vi "SCMP - System init.vi"(8 "error in (no error)":errorcluster, 9 "Pane Color":u32, 10 "instrument":string) -> (0 "error main":errorcluster, 1 "Andor array":T1[](array[typedef]) {"Exposure (s)" format="%^.3g"; "Time at Synch" format="%<%H:%M:%S>T"; "Interframe Time" format="%#_3g"; "Frame Readout Time" format="%_3g"; "Row Readout Time" format="%_3g"}, 2 "Peripherals":T4, 3 "cont?":bool=TRUE, 5 "Today's SCMP Engineering File":path, 7 "version":string)   [LabVIEW 2014]
uses:
  Controls/Global demo.vi
  AISAS/Controls/focus.ctl
  Controls/CoMP-S Controls/Emission Line Filter Wheel.ctl
  Controls/CoMP-S Controls/Polarization Optics Filter Wheel.ctl
  Controls/SCD - EDT - Emission Line Filter Wheel.ctl
  Controls/SCD - Calibration Optics Filter Wheel.ctl
  AISAS/Controls/Diffuser.ctl
  Controls/SCD - FITS Cluster.ctl
  Controls/Globals.vi
  AISAS/Mech/AISAS Mech.lvclass
  Controls/peripherals.ctl
  Controls/Cameras select.ctl
  Camera/Andor Neo Info.ctl
  Controls/beaning.ctl
panel:
  in  "Force PI Init":bool
  in  "Shutter":string(combo)="Global"
  in  "Temperature":string(combo)="-25.00"
  out "Andor 2":T1={"Handle"=0, "Pixel Encoding"="", "AOI Width"=0, "AOI Height"=0, "AOI Stride"=0, "Row Readout Time"=0.0, "Frame Readout Time"=0.0, "Interframe Time"=0.0, "Semaphore"=refnum, "SerialNumber"="", "Camera Model"="", "Controller ID"="", "Firmware Version"="", "Shutter"="Global", "BDiv"=1, "Time at Synch"=timestamp(3029526000.379448 s since 1904-01-01), "Idx"=0, "PreAmp"="", "Binning"=enum."1x1", "PixelReadoutRate"="", "Exposure (s)"=0.05, "Image Bytes"=0, "Image Pixels"=0, "SpuriousNoiseFilter"=FALSE, "Overlap"=FALSE, "CycleMode"=""} {"Exposure (s)" format="%^.3g"; "Time at Synch" format="%<%H:%M:%S>T"; "Interframe Time" format="%#_3g"; "Frame Readout Time" format="%_3g"; "Row Readout Time" format="%_3g"}
  out "Timestamp at Synch 2":timestamp
  out "error eng":errorcluster
  out "Andor 1":T1={"Handle"=0, "Pixel Encoding"="", "AOI Width"=0, "AOI Height"=0, "AOI Stride"=0, "Row Readout Time"=0.0, "Frame Readout Time"=0.0, "Interframe Time"=0.0, "Semaphore"=refnum, "SerialNumber"="", "Camera Model"="", "Controller ID"="", "Firmware Version"="", "Shutter"="Global", "BDiv"=1, "Time at Synch"=timestamp(3029526000.379448 s since 1904-01-01), "Idx"=0, "PreAmp"="", "Binning"=enum."1x1", "PixelReadoutRate"="", "Exposure (s)"=0.05, "Image Bytes"=0, "Image Pixels"=0, "SpuriousNoiseFilter"=FALSE, "Overlap"=FALSE, "CycleMode"=""} caption="Andor1" {"Exposure (s)" format="%^.3g"; "Time at Synch" format="%<%H:%M:%S>T"; "Interframe Time" format="%#_3g"; "Frame Readout Time" format="%_3g"; "Row Readout Time" format="%_3g"}
  out "Timestamp at Synch":timestamp
  # "System initialization\n        wait please"
  # "Peripherals"
  # "Andor control"
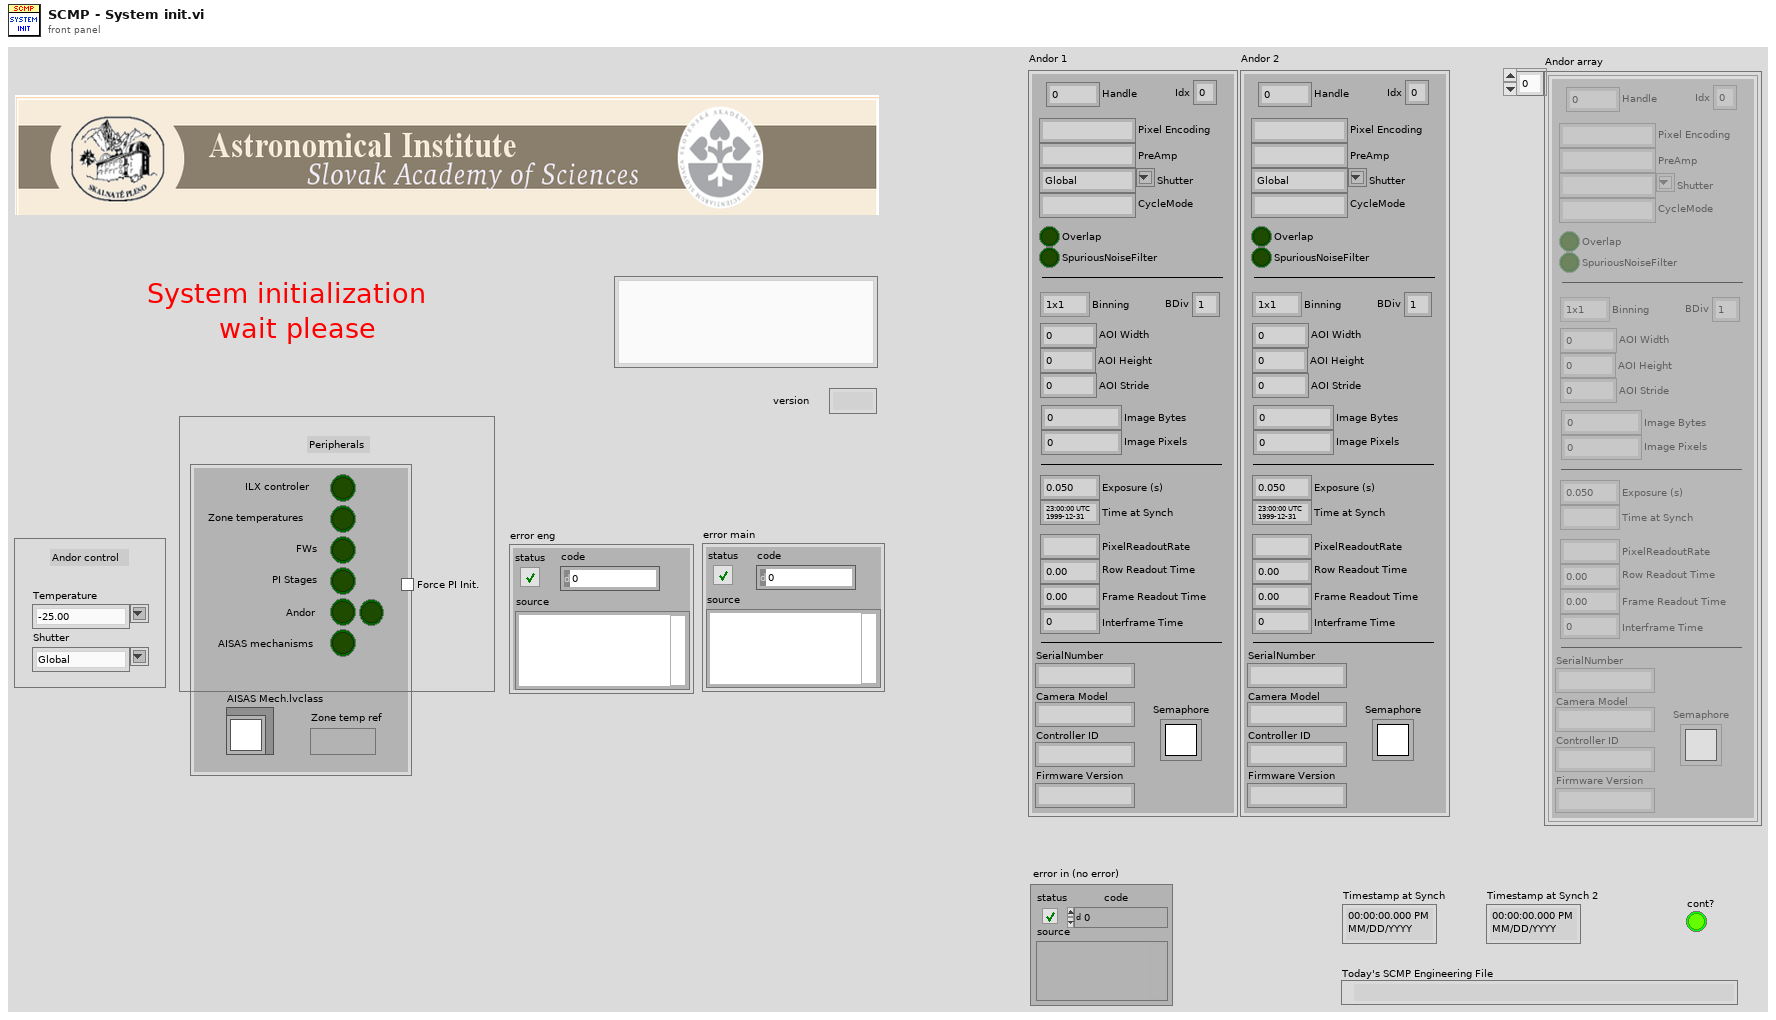
[diagram p1: front panel]
types:
  T1 = typedef "Andor Neo Info.ctl" = cluster{"Handle":i32, "Pixel Encoding":string, "AOI Width":i32, "AOI Height":i32, "AOI Stride":i32, "Row Readout Time":dbl, "Frame Readout Time":dbl, "Interframe Time":dbl, "Semaphore":T2, "SerialNumber":string, "Camera Model":string, "Controller ID":string, "Firmware Version":string, "Shutter":string, "BDiv":u8, "Time at Synch":timestamp, "Idx":i32, "PreAmp":string, "Binning":T3, "PixelReadoutRate":string, "Exposure (s)":dbl, "Image Bytes":i64, "Image Pixels":i64, "SpuriousNoiseFilter":bool, "Overlap":bool, "CycleMode":string}
  T2 = typedef "Semaphore RefNum" = refnum<k1>
  T3 = typedef "beaning.ctl" = enum16{"1x1", "2x2", "3x3", "4x4", "8x8"}
  T4 = typedef "peripherals.ctl" = cluster{"ILX controler":bool, "Zone temperatures":bool, "Andor":bool, "Andor 2":bool, "PI Stages":bool, "AISAS mechanisms":bool, "AISAS Mech.lvclass":refnum<class "AISAS Mech.lvclass">, "Zone temp ref":variant, "FWs":bool}
  T5 = cluster{"server address":string, "remote port (502)":u16}
  T6 = enum32{"Invalid", "Standard", "Closed", "Hidden", "Minimized", "Maximized"}
  T7 = typedef "SCD - FITS Cluster.ctl" = cluster{"Wavelength (nm)":dbl, "Exposure (s)":dbl, "Tuning Delay (ms)":dbl, "Beam Type (-1/1)":dbl, "Tuning Voltages":dbl[], "Observer":string, "Light Shapping Diffuser":T8, "Comment":string, "Data Type":u16, "Mod Cycles":u16, "SCD Calibration Optics":T9, "SCD Emission Line Filter":T10, "Cookbook":string, "COMP-S Calibration Wheel":T11, "COMP-S Andover Filter Wheel":T12, "FOV Rotation (deg)":dbl, "Objective Lens Position (mm)":T13, "Occulter size":dbl, "Time End":timestamp, "Acc Exposure (s)":dbl, "Time Stamp Array":timestamp[], "Camera Serial Number":string[], "Camera Temp":dbl[], "Camera PI (mm)":dbl[], "Time Start":timestamp, "Peripherals":T4, "FITS paths":path[], "Cameras":T14, "load preset cbk":bool, "periodic check count":i32, "COMP-S Calibration Wheel 2":T11, "Calib":enum16{"Dark", "Flat"}, "Abso Aperture":dbl, "Nominal Aperture":dbl}
  T8 = typedef "Diffuser.ctl" = enum16{"Out of Beam", "In Beam"}
  T9 = typedef "SCD - Calibration Optics Filter Wheel.ctl" = enum16{"1 - Polarizer @0, I+Q", "2 - Polarizer @90, I-Q", "3 - Polarizer @45, I+U", "4 - Polarizer @135, I-U", "5 - Polarizer @0, Retarder @45, I+V", "6 - Polarizer @0, Retarder @135, I-V", "7 - Dark", "8 - Clear", "9 - N/A"}
  T10 = typedef "SCD - EDT - Emission Line Filter Wheel.ctl" = enum16{"1-557.6nm", "2-587.6nm", "3-589.6nm", "4-630.2nm", "5-656.4nm", "6-849.8nm", "7-854.2nm", "8-866.2nm", "9-1083.0nm"}
  T11 = typedef "Polarization Optics Filter Wheel.ctl" = enum16{"Dark", "Clear", "Exchange Lens", "Polarizer @0, I+Q", "Polarizer @90, I-Q", "Polarizer @45, I+U", "Polarizer @135, I-U", "Polarizer @0, Retarder @45, I+V", "Polarizer @0, Retarder @135, I-V"}
  T12 = typedef "Emission Line Filter Wheel.ctl" = enum16{"530.3nm/HWB 0.34nm (Fe XIV)", "587.6nm/HBW 0.44nm (He I D3)", "637.5nm/HBW 0.53nm (Fe X)", "656.3nm/HBW 0.57nm (H-Alpha)", "789.2nm/HBW 0.85nm (Fe XI)", "854.2nm/HBW 1.01nm (Ca I)", "1074.7nm/HBW 2.34nm (Fe XIII)", "1079.8nm/HBW 1.64nm (Fe XIII)", "1083.0nm/HBW 1.66nm (He I)"}
  T13 = typedef "focus.ctl" = dbl
  T14 = typedef "Cameras select.ctl" = enum16{"Andor", "GDR"}
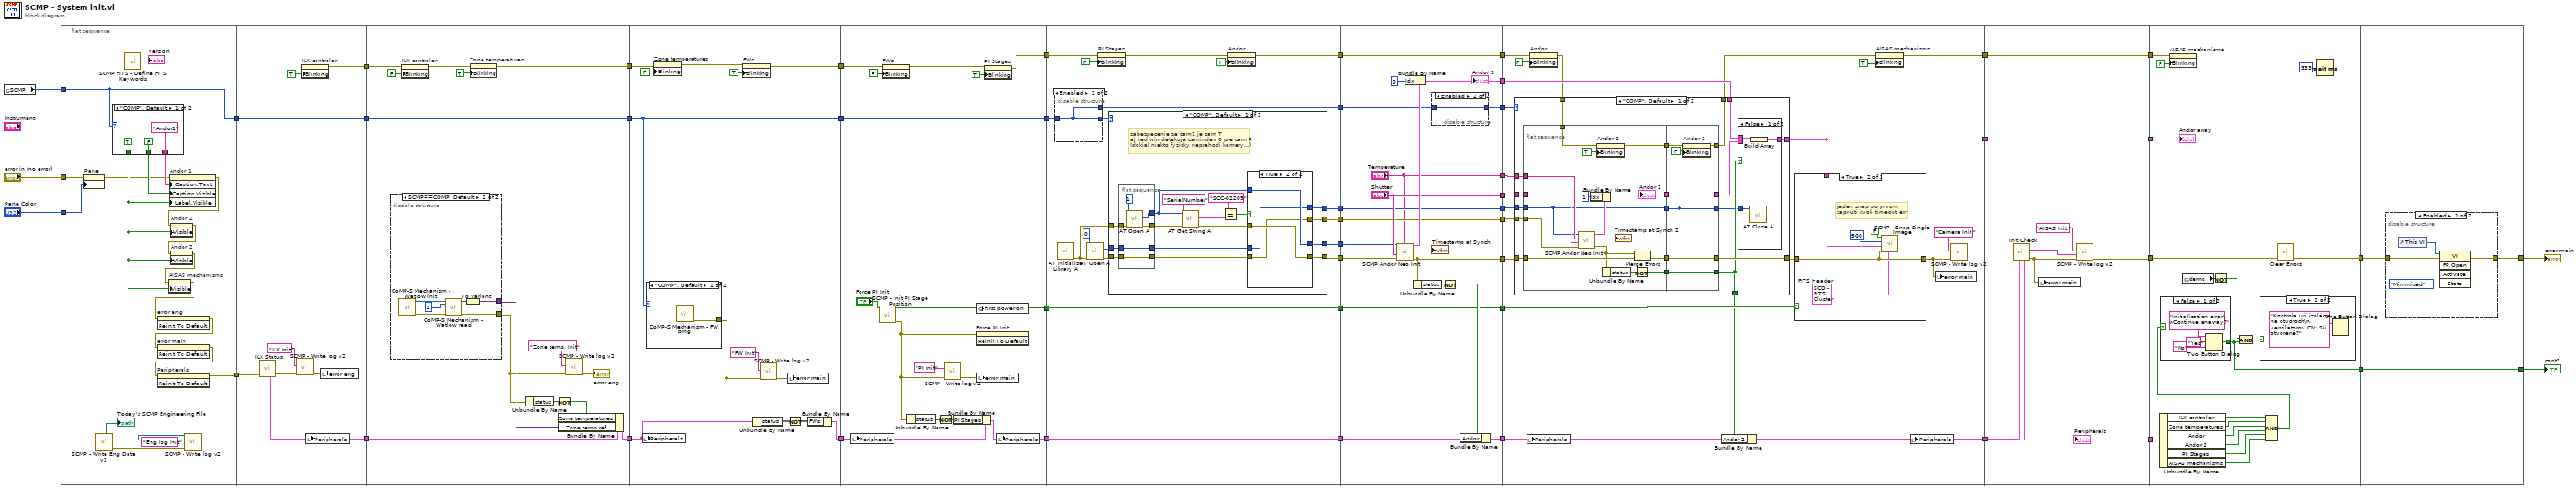
[diagram p0: block diagram]
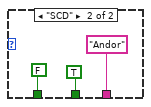
[diagram p2: hidden frame]
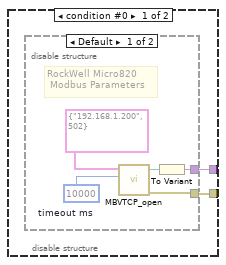
[diagram p3: hidden frame]
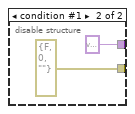
[diagram p4: hidden frame]
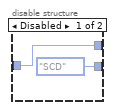
[diagram p6: hidden frame]
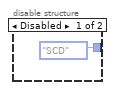
[diagram p9: hidden frame]
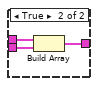
[diagram p10: hidden frame]
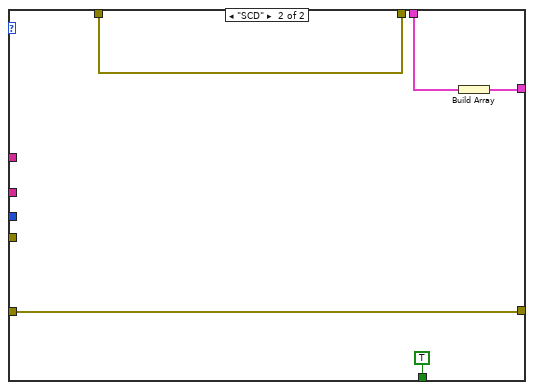
[diagram p11: hidden frame]
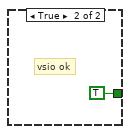
[diagram p14: hidden frame]
diagram:
  n1 = global read "Globals.vi" "SCMP"() -> (w11:enum16{"COMP", "SCD"})
  n2 = flat-sequence {
    tunnel: [w61] -> w38
    tunnel: [w53] -> w19
    tunnel: "error in (no error)" -> [w56]
    tunnel: "Pane Color" -> [w54]
    tunnel: w11 -> [w53]
    tunnel: [w73] -> w8
    tunnel: [w79] -> w7
    tunnel: w38 -> [w78]
    tunnel: w19 -> [w77]
    tunnel: [w77] -> w6
    tunnel: w8 -> [w92]
    tunnel: [w91] -> w41
    tunnel: [w89] -> w39
    tunnel: [w87] -> w16
    tunnel: w6 -> [w87]
    tunnel: w7 -> [w85]
    tunnel: w41 -> [w115]
    tunnel: [w116] -> w40
    tunnel: w39 -> [w120]
    tunnel: [w114] -> w17
    tunnel: w16 -> [w114]
    tunnel: [w117] -> w5
    tunnel: w40 -> [w130]
    tunnel: [w136] -> w29
    tunnel: [w131] -> w18
    tunnel: w17 -> [w131]
    tunnel: w5 -> [w127]
    tunnel: [w125] -> w4
    tunnel: [w123] -> w3
    tunnel: [w143] -> w37
    tunnel: [w152] -> w36
    tunnel: [w149] -> w33
    tunnel: [w148] -> w32
    tunnel: [w147] -> w31
    tunnel: [w146] -> w30
    tunnel: w29 -> [w144]
    tunnel: [w144] -> w28
    tunnel: w18 -> [w139]
    tunnel: w4 -> [w141]
    tunnel: w3 -> [w143]
    tunnel: [w138] -> w2
    tunnel: [w209] -> w47
    tunnel: [w201] -> w46
    tunnel: [w206] -> w45
    tunnel: ["Shutter"] -> w44
    tunnel: ["Temperature"] -> w43
    tunnel: w37 -> [w204]
    tunnel: [w200] -> w42
    tunnel: w36 -> [w200]
    tunnel: [w196] -> w35
    tunnel: [w197] -> w34
    tunnel: w33 -> [w199]
    tunnel: w32 -> [w198]
    tunnel: w31 -> [w197]
    tunnel: w30 -> [w196]
    tunnel: w28 -> [w195]
    tunnel: [w195] -> w27
    tunnel: [w192] -> w15
    tunnel: w2 -> [w191]
    tunnel: w47 -> [w232]
    tunnel: w46 -> [w222]
    tunnel: [w219] -> w24
    tunnel: w45 -> [w228]
    tunnel: w44 -> [w230]
    tunnel: w43 -> [w229]
    tunnel: w42 -> [w227]
    tunnel: [w221] -> w23
    tunnel: w35 -> [w225]
    tunnel: w34 -> [w224]
    tunnel: w27 -> [w223]
    tunnel: [w214] -> w20
    tunnel: w15 -> [w212]
    tunnel: [w297] -> w25
    tunnel: w24 -> [w292]
    tunnel: w23 -> [w298]
    tunnel: [w298] -> w22
    tunnel: [w296] -> w21
    tunnel: w20 -> [w296]
    tunnel: [w291] -> w14
    tunnel: w25 -> [w300]
    tunnel: w22 -> [w315]
    tunnel: w21 -> [w313]
    tunnel: w14 -> [w301]
    tunnel: [w299] -> w10
    tunnel: [w304] -> w9
    tunnel: [w325] -> w26
    tunnel: w10 -> [w324]
    tunnel: w9 -> [w325]
    tunnel: [w323] -> w1
    frame #0 {
      n3 = property on="Pane" class="Pane"(error in=w56, "PaneColor"=w54) -> (error out=w55:errorcluster)  [unwired: 1 in, 1 out]
      n4 = call "SCMP - Write Eng Data v2.vi"() -> ("error out"=w48:errorcluster, "Today's SCMP folder"=w51:path, "Today's SCMP Engineering File"=→"Today's SCMP Engineering File":path)  [unwired: 8 in, 1 out]
      n5 = case shown="\"COMP\", Default" w53 {
        tunnel: ["Andor1" ("Caption.Text") "Andor" ("Caption.Text")] -> w66
        tunnel: [FALSE ("Caption.Visible") TRUE ("Caption.Visible")] -> w65
        tunnel: [TRUE ("Caption.Visible") FALSE ("Caption.Visible")] -> w58
        frame "COMP", Default {
        }
        frame "SCD" {
        }
      }
      n6 = call "SCMP FITS - Define FITS Keywords.vi"() -> ("Version"=→"version":string)  [unwired: 5 in, 6 out]
      n7 = property on="Andor 1" class="Clust (strict)"(error in=w55, "Caption.Text"=w66, "Caption.Visible"=w65, "Label.Visible"=w58) -> (error out=w64:errorcluster)  [unwired: 1 in, 1 out]
      n8 = property on="Andor 2" class="Clust (strict)"(error in=w64, "Visible"=w58) -> (error out=w60:errorcluster)  [unwired: 1 in, 1 out]
      n9 = property on="Andor 2" class="Bool (strict)"(error in=w60, "Visible"=w58) -> (error out=w59:errorcluster)  [unwired: 1 in, 1 out]
      n10 = property on="AISAS mechanisms" class="Bool (strict)"(error in=w59, "Visible"=w58) -> (error out=w57:errorcluster)  [unwired: 1 in, 1 out]
      n11 = invoke on="error eng" class="Clust (strict)" method="Reinit To Default"(error in=w57) -> (error out=w63:errorcluster)  [unwired: 2 in, 2 out]
      n12 = invoke on="error main" class="Clust (strict)" method="Reinit To Default"(error in=w63) -> (error out=w62:errorcluster)  [unwired: 2 in, 2 out]
      n13 = invoke on="Peripherals" class="Clust (strict)" method="Reinit To Default"(error in=w62) -> (error out=w61:errorcluster)  [unwired: 2 in, 2 out]
      n14 = call "SCMP - Write log v2.vi"("Error to log"=w48, "data"="Eng log Init" ("mesage"), "Today's SCMP folder"=w51) -> ()  [unwired: 6 in, 3 out]
    }
    frame #1 {
      n15 = call "ILX Status.vi"("error in"=w78) -> ("error out"=w76:errorcluster, "Peripherals out"=w73:T4)  [unwired: 5 in, 4 out]
      n16 = call "SCMP - Write log v2.vi"("Error to log"=w76, "data"="ILX Init" ("mesage")) -> ("error out"=w74:errorcluster)  [unwired: 7 in, 2 out]
      n17 = property on="ILX controler" class="Bool (strict)"("Blinking"=TRUE) -> (error out=w79:errorcluster)  [unwired: 2 in, 1 out]
      n18 = local write "Peripherals"(w73) -> ()
      n19 = local write "error eng"(w74) -> ()
    }
    frame #2 {
      n20 = disable-structure shown="SCMP==COMP, Default" {
        disable-tunnel: [w96 w104] -> w82
        disable-tunnel: [w95 w105] -> w88
        frame condition #0 {
          n21 = disable-structure shown="Default" {
            disable-tunnel: [w97 errorcluster {"status"=FALSE, "code"=0, "source"=""} ("error in")] -> w96
            disable-tunnel: [w98 variant ("Variant")] -> w95
            frame condition #0 (active) {
              w100 = 10000  # timeout ms
              # "RockWell Micro820\n Modbus Parameters"
              n22 = call <vilib>:"MBVTCP_open.vi"("timeout ms (60000)"=w100, "Network"=T5 {"server address"="192.168.1.200", "remote port (502)"=502} ("Rockwell Address and Port")) -> ("error out"=w97:errorcluster, "NetRefTCP out"=w99:refnum<k5>)  [unwired: 1 in, 7 out]
              n23 = To Variant(anything=w99) -> (Variant=w98:variant)
            }
            frame condition #1 {
            }
          }
        }
        frame condition #1 (active) {
          n24 = call "CoMP-S Mechanism - Watlow init.vi"() -> ("error out"=w106:errorcluster, "ILabVIEW"=w107:refnum<k24>)  [unwired: 8 in, 1 out]
          n25 = call "CoMP-S Mechanism - Watlow read.vi"("6. Instance ID"=1, "error in (no error)"=w106, "ILabVIEW In"=w107) -> ("error out"=w104:errorcluster)  [unwired: 4 in, 2 out]
          n26 = To Variant(anything=w107) -> (Variant=w105:variant)
        }
      }
      n27 = property on="ILX controler" class="Bool (strict)"(error in=w85, "Blinking"=FALSE) -> (error out=w84:errorcluster)  [unwired: 1 in, 1 out]
      n28 = property on="Zone temperatures" class="Bool (strict)"(error in=w84, "Blinking"=TRUE) -> (error out=w89:errorcluster)  [unwired: 1 in, 1 out]
      n29 = Unbundle By Name(w82) -> ("status"=w94:bool)
      n30 = Not(x=w94) -> (.not. x?=w90:bool)
      n31 = Bundle By Name(cluster=w92, "Zone temperatures"=w90, "Zone temp ref"=w88) -> (w91:T4)
      n32 = call "SCMP - Write log v2.vi"("Error to log"=w82, "data"="Zone temp. Init" ("mesage")) -> ("error out"=→"error eng":errorcluster)  [unwired: 7 in, 2 out]
    }
    frame #3 {
      n33 = local write "Peripherals"(w115) -> ()
      n34 = case shown="\"COMP\", Default" w114 {
        tunnel: [w122 _] -> w111
        frame "COMP", Default {
          n35 = call "CoMP-S Mechanism - FW ping.vi"() -> ("error out"=w122:errorcluster)  [unwired: 10 in, 1 out]
        }
        frame "SCD" {
        }
      }
      n36 = property on="Zone temperatures" class="Bool (strict)"(error in=w120, "Blinking"=FALSE) -> (error out=w118:errorcluster)  [unwired: 1 in, 1 out]
      n37 = property on="FWs" class="Bool (strict)"(error in=w118, "Blinking"=TRUE) -> (error out=w117:errorcluster)  [unwired: 1 in, 1 out]
      n38 = Unbundle By Name(w111) -> ("status"=w113:bool)
      n39 = call "SCMP - Write log v2.vi"("Error to log"=w111, "data"="FW Init" ("mesage")) -> ("error out"=w109:errorcluster)  [unwired: 7 in, 2 out]
      n40 = Not(x=w113) -> (.not. x?=w112:bool)
      n41 = local write "error main"(w109) -> ()
      n42 = Bundle By Name(cluster=w115, "FWs"=w112) -> (w116:T4)
    }
    frame #4 {
      n43 = local write "Peripherals"(w130) -> ()
      n44 = call "SCMP - Init PI Stage Position.vi"("Force PI Init"="Force PI Init") -> ("error out"=w124:errorcluster, "first power on"=w136:bool)  [unwired: 9 in]
      n45 = property on="FWs" class="Bool (strict)"(error in=w127, "Blinking"=FALSE) -> (error out=w126:errorcluster)  [unwired: 1 in, 1 out]
      n46 = Unbundle By Name(w124) -> ("status"=w135:bool)
      n47 = Not(x=w135) -> (.not. x?=w134:bool)
      n48 = call "SCMP - Write log v2.vi"("Error to log"=w124, "data"="PI Init" ("mesage")) -> ("error out"=w132:errorcluster)  [unwired: 7 in, 2 out]
      n49 = Bundle By Name(cluster=w130, "PI Stages"=w134) -> (w123:T4)
      n50 = global write "Globals.vi" "first power on"(w136) -> ()
      n51 = invoke on="Force PI Init" class="Bool (strict)" method="Reinit To Default"(error in=w124) -> ()  [unwired: 2 in, 3 out]
      n52 = local write "error main"(w132) -> ()
      n53 = property on="PI Stages" class="Bool (strict)"(error in=w126, "Blinking"=TRUE) -> (error out=w125:errorcluster)  [unwired: 1 in, 1 out]
      n54 = local write "Peripherals"(w123) -> ()
    }
    frame #5 {
      n55 = disable-structure shown="Enabled" {
        disable-tunnel: [enum16{"COMP", "SCD"}."SCD" ("SCMP") w158] -> w140
        disable-tunnel: w139 -> [w156 w158]
        disable-tunnel: [w156 w158] -> w138
        frame Disabled {
        }
        frame Enabled {
        }
      }
      n56 = call <userlib>:"AT Initialise Library A.vi"() -> ("error out"=w142:errorcluster)  [unwired: 10 in, 1 out]
      n57 = call <userlib>:"AT Open A.vi"("error in (no error)"=w142, "CameraIndex"=0) -> ("error out"=w150:errorcluster, "Handle"=w145:i32)  [unwired: 7 in, 1 out]
      n58 = property on="PI Stages" class="Bool (strict)"(error in=w141, "Blinking"=FALSE) -> (error out=w155:errorcluster)  [unwired: 1 in, 1 out]
      n59 = case shown="\"COMP\", Default" w140 {
        tunnel: w150 -> [w174 w189]
        tunnel: [w173 w190] -> w149
        tunnel: [w172 w189] -> w148
        tunnel: [w171 _] -> w147
        tunnel: [w170 _] -> w146
        tunnel: w145 -> [w169 w190]
        tunnel: w142 -> [w168 _]
        frame "COMP", Default {
          # "zabezpecenie ze cam1 je cam T\naj ked win detekuje camindex 0 pre cam R\n(dokial niekto fyzicky neprehodi kamery...)"
          n60 = flat-sequence {
            tunnel: w174 -> [w186]
            tunnel: [w187] -> w166
            tunnel: [w184] -> w159
            tunnel: w169 -> [w185]
            tunnel: [w186] -> w161
            tunnel: [w185] -> w160
            tunnel: w168 -> [w183]
            frame #0 {
              n61 = call <userlib>:"AT Open A.vi"("error in (no error)"=w183, "CameraIndex"=1) -> ("error out"=w187:errorcluster, "Handle"=w184:i32)  [unwired: 7 in, 1 out]
            }
          }
          n62 = call <userlib>:"AT Get String A.vi"("error in (no error)"=w166, "Feature"="SerialNumber", "Handle"=w159) -> ("error out"=w162:errorcluster, "String"=w165:string)  [unwired: 6 in, 1 out]
          n63 = Equal?(x="SCC-02209", y=w165) -> (x = y?=w163:bool)
          n64 = case shown="True" w163 {
            tunnel: w162 -> [w176 w181]
            tunnel: w161 -> [w178 w179]
            tunnel: w160 -> [w177 w180]
            tunnel: w159 -> [w175 w182]
            tunnel: [w177 w182] -> w173
            tunnel: [w178 w181] -> w172
            tunnel: [w175 w180] -> w171
            tunnel: [w176 w179] -> w170
            frame False {
            }
            frame True {
            }
          }
        }
        frame "SCD" {
        }
      }
      n65 = property on="Andor" class="Bool (strict)"(error in=w155, "Blinking"=TRUE) -> (error out=w152:errorcluster)  [unwired: 1 in, 1 out]
    }
    frame #6 {
      n66 = call "SCMP Andor Neo Init.vi"("error in"=w198, "Shutter"="Shutter", "Temperature"="Temperature", "Neo Handle"=w199) -> ("error out"=w209:errorcluster, "Timestamp at Synch"=→"Timestamp at Synch":timestamp, "Neo Info"=w207:T1)  [unwired: 5 in]
      n67 = Bundle By Name(cluster=w207, "Idx"=0 ("CameraIndex")) -> (w201:T1)
      "Andor 1" <- w201
      n68 = Unbundle By Name(w209) -> ("status"=w208:bool)
      n69 = disable-structure shown="Enabled" {
        disable-tunnel: [enum16{"COMP", "SCD"}."SCD" ("SCMP") w211] -> w192
        disable-tunnel: w191 -> [_ w211]
        frame Disabled {
        }
        frame Enabled {
        }
      }
      n70 = Not(x=w208) -> (.not. x?=w203:bool)
      n71 = Bundle By Name(cluster=w204, "Andor"=w203) -> (w206:T4)
    }
    frame #7 {
      n72 = local write "Peripherals"(w228) -> ()
      n73 = property on="Andor" class="Bool (strict)"(error in=w227, "Blinking"=FALSE) -> (error out=w217:errorcluster)  [unwired: 1 in, 1 out]
      n74 = case shown="\"COMP\", Default" w212 {
        tunnel: w232 -> [w245 w283]
        tunnel: w230 -> [w244 _]
        tunnel: w229 -> [w243 _]
        tunnel: [w242 w283] -> w226
        tunnel: w225 -> [w241 _]
        tunnel: w224 -> [w240 _]
        tunnel: w222 -> [w239 w281]
        tunnel: [w238 w280] -> w221
        tunnel: w217 -> [w237 w284]
        tunnel: [w236 w284] -> w215
        tunnel: [w235 TRUE] -> w213
        frame "COMP", Default {
          n75 = flat-sequence {
            tunnel: [w270] -> w250
            tunnel: w245 -> [w271]
            tunnel: [w264] -> w249
            tunnel: w244 -> [w266]
            tunnel: w243 -> [w261]
            tunnel: w241 -> [w263]
            tunnel: w240 -> [w257]
            tunnel: w237 -> [w260]
            tunnel: [w259] -> w248
            tunnel: [w258] -> w247
            tunnel: [w257] -> w246
            tunnel: [w277] -> w242
            tunnel: w250 -> [w277]
            tunnel: [w279] -> w234
            tunnel: w249 -> [w279]
            tunnel: w248 -> [w276]
            tunnel: [w275] -> w236
            tunnel: w247 -> [w274]
            tunnel: [w274] -> w235
            tunnel: w246 -> [w273]
            tunnel: [w273] -> _
            tunnel: [w273] -> w233
            frame #0 {
              n76 = call "SCMP Andor Neo Init.vi"("error in"=w263, "Shutter"=w266, "Temperature"=w261, "Neo Handle"=w257) -> ("error out"=w269:errorcluster, "Timestamp at Synch"=→"Timestamp at Synch 2":timestamp, "Neo Info"=w268:T1)  [unwired: 5 in]
              n77 = Bundle By Name(cluster=w268, "Idx"=1 ("CameraIndex")) -> (w264:T1)
              "Andor 2" <- w264
              n78 = property on="Andor 2" class="Bool (strict)"(error in=w260, "Blinking"=TRUE) -> (error out=w259:errorcluster)  [unwired: 1 in, 1 out]
              n79 = Unbundle By Name(w269) -> ("status"=w272:bool)
              n80 = Not(x=w272) -> (.not. x?=w258:bool)
              n81 = Merge Errors(w269, w271) -> (w270:errorcluster)
            }
            frame #1 {
              n82 = property on="Andor 2" class="Bool (strict)"(error in=w276, "Blinking"=FALSE) -> (error out=w275:errorcluster)  [unwired: 1 in, 1 out]
            }
          }
          n83 = case shown="False" w235 {
            tunnel: [w253 w256] -> w238
            tunnel: w239 -> [w252 w255]
            tunnel: w234 -> [_ w254]
            tunnel: w233 -> [w251 _]
            frame False {
              n84 = call <userlib>:"AT Close A.vi"("Handle"=w251) -> ()  [unwired: 9 in, 2 out]
              n85 = Build Array(w252) -> (w253:T1[])
            }
            frame True {
              n86 = Build Array(w255, w254) -> (w256:T1[])
            }
          }
        }
        frame "SCD" {
          n87 = Build Array(w281) -> (w280:T1[])
        }
      }
      n88 = Bundle By Name(cluster=w228, "Andor 2"=w213) -> (w219:T4)
      n89 = case shown="True" w223 {
        tunnel: w226 -> [w285 w288]
        tunnel: [w285 w288] -> w220
        tunnel: w221 -> [_ w287]
        frame False {
        }
        frame True {
          w286 = T7 {"Wavelength (nm)"=0.0, "Exposure (s)"=0.0, "Tuning Delay (ms)"=0.0, "Beam Type (-1/1)"=0.0, "Tuning Voltages"=[], "Observer"="", "Light Shapping Diffuser"=enum."Out of Beam", "Comment"="", "Data Type"=0, "Mod Cycles"=0, "SCD Calibration Optics"=enum."1 - Polarizer @0, I+Q", "SCD Emission Line Filter"=enum."1-557.6nm", "Cookbook"="", "COMP-S Calibration Wheel"=enum."Dark", "COMP-S Andover Filter Wheel"=enum."530.3nm/HWB 0.34nm (Fe XIV)", "FOV Rotation (deg)"=0.0, "Objective Lens Position (mm)"=0.0, "Occulter size"=0.0, "Time End"=timestamp(0 s since 1904-01-01), "Acc Exposure (s)"=0.0, "Time Stamp Array"=[], "Camera Serial Number"=[], "Camera Temp"=[], "Camera PI (mm)"=[], "Time Start"=timestamp(3382374145.421875 s since 1904-01-01), "Peripherals"={"ILX controler"=FALSE, "Zone temperatures"=FALSE, "Andor"=FALSE, "Andor 2"=FALSE, "PI Stages"=FALSE, "AISAS mechanisms"=FALSE, "AISAS Mech.lvclass"=refnum, "Zone temp ref"=variant, "FWs"=FALSE}, "FITS paths"=[], "Cameras"=enum."Andor", "load preset cbk"=FALSE, "periodic check count"=0, "COMP-S Calibration Wheel 2"=enum."Dark", "Calib"=enum."Dark", "Abso Aperture"=40.0, "Nominal Aperture"=196.0}  # FITS Header
          # "jeden snap po prvom \nzapnuti kvoli timeout err"
          n90 = call "SCMP - Snap Single Image.vi"("FITS Header"=w286, "error in"=w288, "Andor Neo"=w287, "Timeout"=u32 500, "Save Data to FITS? (F)"=FALSE) -> ()  [unwired: 2 in, 5 out]
        }
      }
      n91 = property on="AISAS mechanisms" class="Bool (strict)"(error in=w215, "Blinking"=TRUE) -> (error out=w214:errorcluster)  [unwired: 1 in, 1 out]
      n92 = local write "Peripherals"(w219) -> ()
      n93 = local write "error main"(w220) -> ()
      n94 = call "SCMP - Write log v2.vi"("Error to log"=w220, "data"="Camera Init ") -> ()  [unwired: 7 in, 3 out]
    }
    frame #8 {
      n95 = call "Init Check.vi"("Peripherals in"=w292) -> ("error out"=w295:errorcluster, "auto off resp"=w293:string, "Peripherals out"=w291:T4)  [unwired: 7 in, 1 out]
      "Peripherals" <- w291
      n96 = local write "error main"(w295) -> ()
      n97 = call "SCMP - Write log v2.vi"("Error to log"=w295, "data to end"=w293, "data"="AISAS Init ") -> ("error out"=w297:errorcluster)  [unwired: 6 in, 2 out]
    }
    frame #9 {
      n98 = Unbundle By Name(w301) -> ("ILX controler"=w312:bool, "Zone temperatures"=w311:bool, "Andor"=w310:bool, "Andor 2"=w309:bool, "PI Stages"=w308:bool, "AISAS mechanisms"=w307:bool)
      n99 = property on="AISAS mechanisms" class="Bool (strict)"(error in=w313, "Blinking"=FALSE) -> ()  [unwired: 1 in, 2 out]
      n100 = global read "Global demo.vi" "demo"() -> (w305:bool)
      n101 = Not(x=w305) -> (.not. x?=w302:bool)
      n102 = Compound Arithmetic op=AND(w312, w311, w310, w309, w308, w307) -> (w306:bool)
      n103 = case shown="False" w306 {
        tunnel: [w318 TRUE ("T button?")] -> w304
        frame False {
          n104 = Two Button Dialog(message="Initialization error\nContinue anaway?", 1:"No" ("F button name (\"Cancel\")"), 2:"Yes" ("T button name (\"OK\")")) -> (T button?=w318:bool)
        }
        frame True {
          # "vsio ok"
        }
      }
      n105 = And(x=w302, y=w304) -> (x .and. y?=w303:bool)
      n106 = case shown="True" w303 {
        frame False {
        }
        frame True {
          n107 = One Button Dialog(message="Kontrola uší izolácie na otvoroch\n  ventilátorov CM: Sú otvorené?") -> ()  [unwired: 1 in, 1 out]
        }
      }
      n108 = call <vilib>:"Clear Errors.vi"("error in (no error)"=w300) -> ("error out"=w299:errorcluster)  [unwired: 5 in, 1 out]
      n109 = Wait (ms)(milliseconds to wait=u32 333) -> ()  [unwired: 1 out]
      "Andor array" <- w315
    }
    frame #10 {
      n110 = disable-structure shown="Enabled" {
        disable-tunnel: w324 -> [w327 _]
        disable-tunnel: [w326 _] -> w323
        frame Enabled {
          n111 = control-ref of="This VI"() -> (w328:refnum<vi>)
          n112 = invoke class="VI" method="FP.Open"(reference=w328, error in=w327, "State"=T6."Minimized") -> (error out=w326:errorcluster)  [unwired: 2 in, 4 out]
        }
        frame Disabled {
        }
      }
    }
  }
  "error main" <- w1
  "cont?" <- w26
